vi "WPI_AnalogOutputChannelCache.vi"(7 "Operation":T2, 8 "error in (no error)":errorcluster, 10 "AO Channel":T1) -> (0 "error out":errorcluster, 2 "Allocated?":bool, 3 "Allocated Channel":T1=enum."Invalid")   [LabVIEW 2017]
doc: "This software is licensed. Open the labview\\readme\\WPI Robotics Library Open Source License.txt file for more information."
uses:
  <vilib>/Rock Robotics/WPI/AnalogChannel/WPI_AnalogChannelChannelCacheOp.ctl
  <vilib>/Rock Robotics/WPI/AnalogOutput/WPI_AnalogOutputChannel.ctl
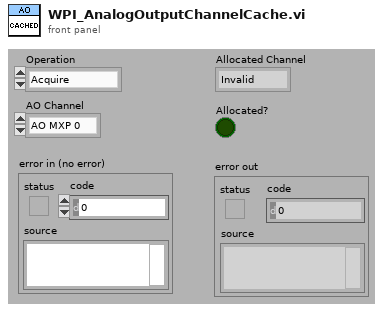
[diagram p1: front panel]
types:
  T1 = typedef "WPI_AnalogOutputChannel.ctl" = enum8{"AO MXP 0", "AO MXP 1", "Invalid"}
  T2 = typedef "WPI_AnalogChannelChannelCacheOp.ctl" = enum16{"Acquire", "Release", "Status"}
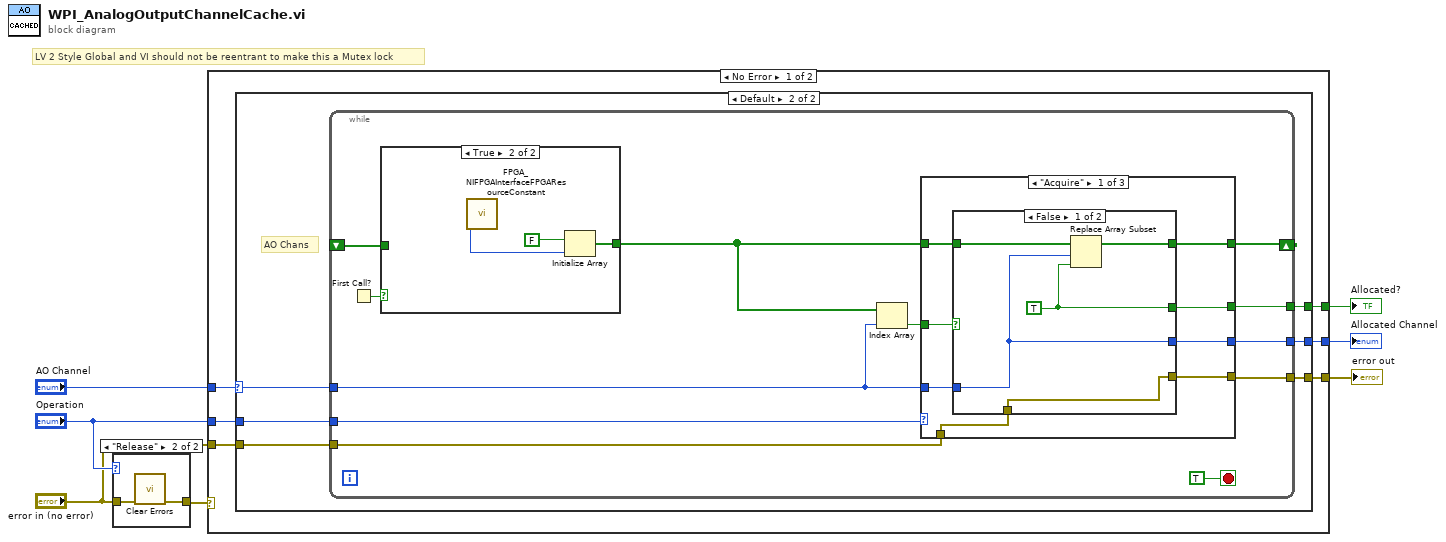
[diagram p0: block diagram]
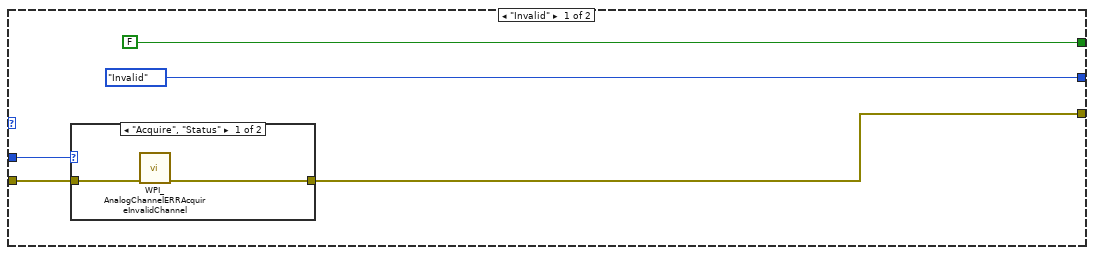
[diagram p3: hidden frame]
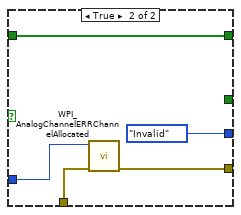
[diagram p5: hidden frame]
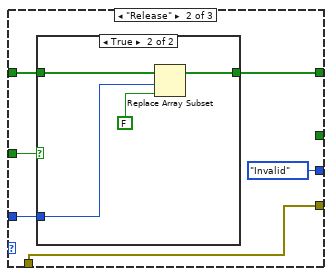
[diagram p6: hidden frame]
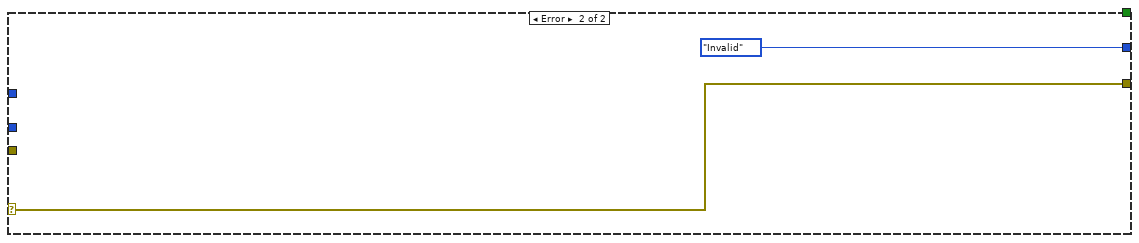
[diagram p10: hidden frame]
diagram:
  # "LV 2 Style Global and VI should not be reentrant to make this a Mutex lock"
  n1 = case shown="\"Release\"" "Operation" {
    tunnel: "error in (no error)" -> [w8 w10]
    tunnel: [w8 w9] -> w6
    frame "Acquire", Default {
    }
    frame "Release" {
      n2 = call <vilib>:"Clear Errors.vi"("error in (no error)"=w10) -> ("error out"=w9:errorcluster)  [unwired: 1 in, 5 out]
    }
  }
  n3 = case shown="No Error" w6 {
    selector: w6 -> [_ w81]
    tunnel: "Operation" -> [w16 _]
    tunnel: "AO Channel" -> [w15 _]
    tunnel: [w14 w81] -> w1
    tunnel: [w13 _] -> w5
    tunnel: [w12 WPI_AnalogOutputChannel."Invalid" ("AO Channel")] -> w4
    tunnel: "error in (no error)" -> [w11 _]
    frame No Error {
      n4 = case shown="Default" w15 {
        selector: w15 -> [_ w26]
        tunnel: w16 -> [w21 w30]
        tunnel: [w20 w29] -> w14
        tunnel: [FALSE ("new element/subarray") w28] -> w13
        tunnel: [WPI_AnalogOutputChannel."Invalid" ("AO Channel") w27] -> w12
        tunnel: w11 -> [w18 w25]
        frame "Invalid" {
          n5 = case shown="\"Acquire\", \"Status\"" w21 {
            tunnel: [w23 w24] -> w20
            tunnel: w18 -> [w22 w24]
            frame "Acquire", "Status" {
              n6 = call <vilib>:"WPI_AnalogChannelERRAcquireInvalidChannel.vi"("error in (no error)"=w22) -> ("error out"=w23:errorcluster)  [unwired: 10 in]
            }
            frame "Release" {
            }
          }
        }
        frame Default {
          # "AO Chans"
          n7 = while {
            shift-right: [w39] -> _
            shift-left: _ -> [w41]
            tunnel: w30 -> [w40]
            tunnel: w26 -> [w35]
            tunnel: [w38] -> w29
            tunnel: [w37] -> w28
            tunnel: [w34] -> w27
            tunnel: w25 -> [w32]
            stop <- TRUE stop-if-true
            n8 = First Call?() -> (First Call?: T/F=w42:bool)
            n9 = case shown="True" w42 {
              tunnel: w41 -> [w76 _]
              tunnel: [w76 w78] -> w36
              frame False {
              }
              frame True {
                n10 = call <vilib>:"FPGA_NIFPGAInterfaceFPGAResourceConstant.vi"() -> ("NumberOfAOChannels"=w77:u8)  [unwired: 11 out]
                n11 = Initialize Array(FALSE, w77) -> (w78:bool[])
              }
            }
            n12 = Index Array(array=w36, index=w35) -> (element=w31:bool)
            n13 = case shown="\"Acquire\"" w40 {
              tunnel: w36 -> [w46 w66 w73]
              tunnel: [w50 w64 w73] -> w39
              tunnel: w35 -> [w49 w65 w75]
              tunnel: [w48 w62 w72] -> w38
              tunnel: [w47 _ w74] -> w37
              tunnel: w31 -> [w45 w63 w74]
              tunnel: [w44 WPI_AnalogOutputChannel."Invalid" ("AO Channel") w75] -> w34
              tunnel: w32 -> [w43 w62 w72]
              frame "Acquire" {
                n14 = case shown="False" w45 {
                  tunnel: w46 -> [w54 w60]
                  tunnel: [w53 w60] -> w50
                  tunnel: w49 -> [w52 w56]
                  tunnel: [w51 w59] -> w48
                  tunnel: [w55 _] -> w47
                  tunnel: [w52 WPI_AnalogOutputChannel."Invalid" ("AO Channel")] -> w44
                  tunnel: w43 -> [w51 w57]
                  frame False {
                    w55 = TRUE ("new element/subarray")
                    n15 = Replace Array Subset(array=w54, new element=w55, index=w52) -> (w53:bool[])
                  }
                  frame True {
                    n16 = call <vilib>:"WPI_AnalogChannelERRChannelAllocated.vi"("error in (no error)"=w57, "AO Channel"=w56) -> ("ERRChannelAllocated"=w59:errorcluster)  [unwired: 9 in]
                  }
                }
              }
              frame "Release" {
                n17 = case shown="True" w63 {
                  tunnel: w66 -> [w67 w71]
                  tunnel: w65 -> [_ w70]
                  tunnel: [w67 w69] -> w64
                  frame False {
                  }
                  frame True {
                    n18 = Replace Array Subset(array=w71, new element=FALSE ("new element/subarray"), index=w70) -> (w69:bool[])
                  }
                }
              }
              frame "Status" {
              }
            }
          }
        }
      }
    }
    frame Error {
    }
  }
  "error out" <- w1
  "Allocated?" <- w5
  "Allocated Channel" <- w4
